vi "Sequential move.vi"(8 "milliseconds to wait":u32, 9 "ENUM":u16[](array[numeric]), 10 "D":dbl) -> ()   [LabVIEW 2017]
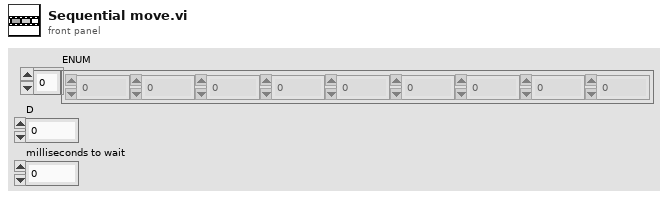
[diagram p1: front panel]
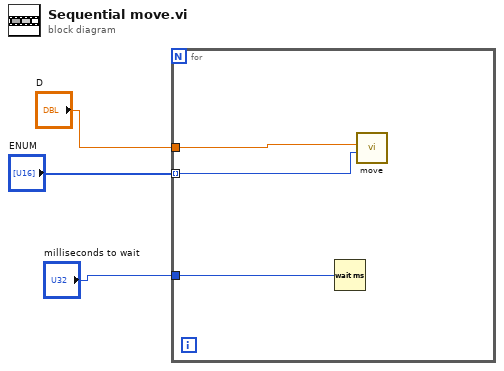
[diagram p0: block diagram]
diagram:
  n1 = for {
    tunnel: "D" -> [w6]
    tunnel: "milliseconds to wait" -> [w5]
    tunnel: "ENUM" -> [w4] mode=indexing
    n2 = Wait (ms)(milliseconds to wait=w5) -> ()  [unwired: 1 out]
    n3 = call "move.vi"("Enum"=w4, "D"=w6) -> ()  [unwired: 10 in]
  }
